vi "Get Byte Count.vi"(8 "error in (no error)":errorcluster, 11 "RFFE Extended Command in":refnum<class "RFFE Extended Command.lvclass">) -> (0 "error out":errorcluster, 2 "Byte Count":i32, 3 "RFFE Extended Command out":refnum<class "RFFE Extended Command.lvclass">)   [LabVIEW 2018, in "MIPI RFFE API.lvlib" / "RFFE Extended Command.lvclass"]
uses:
  RFFE Extended Command.lvclass
  C:/Users/semoore/Projects/mipi-rffe-labview-oop/Command/RFFE Command.lvclass
  Command/RFFE Command.lvclass
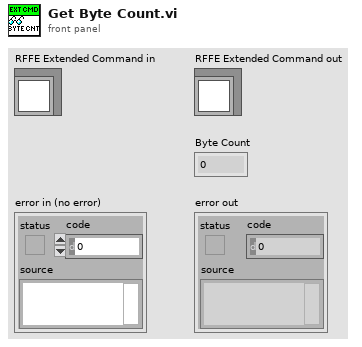
[diagram p1: front panel]
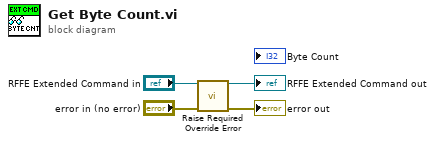
[diagram p0: block diagram]
diagram:
  n1 = call "Raise Required Override Error.vi"("RFFE Command in"="RFFE Extended Command in", "error in (no error)"="error in (no error)") -> ("RFFE Command out"=→"RFFE Extended Command out":refnum<class "RFFE Extended Command.lvclass">, "error out"=→"error out":errorcluster)  [unwired: 11 in, 1 out]
